vi "NewBombedWall.vi"(8 "error in (no error)":errorcluster, 11 "Bomb":bool) -> (0 "error out":errorcluster, 3 "BombedWall":refnum<class "BombedWall.lvclass">)   [LabVIEW 2020, in "BombedWall.lvclass"]
uses:
  BombedWall.lvclass
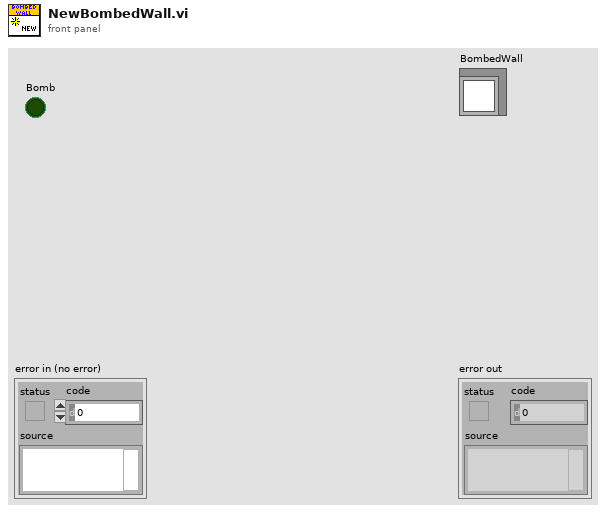
[diagram p1: front panel]
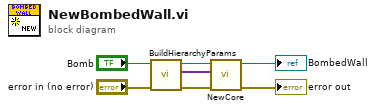
[diagram p0: block diagram]
diagram:
  n1 = call "BuildHierarchyParams.vi"("error in (no error)"="error in (no error)", "Bomb"="Bomb") -> ("error out"=w7:errorcluster, "HierarchyParams"=w6:variant[], "BombedWall"=w5:refnum<class "BombedWall.lvclass">)  [unwired: 7 in]
  n2 = call-dynamic "NewCore.vi"("error in (no error)"=w7, "ParamsArray"=w6, "BombedWall"=w5) -> ("error out"=→"error out":errorcluster, "BombedWall"=→"BombedWall":refnum<class "BombedWall.lvclass">)  [unwired: 7 in]
